vi "main.vi"() -> ()   [LabVIEW 2012]
uses:
  <userlib>/atmcd32d.llb/Error Code Enum typedef.ctl
  <userlib>/atmcd32d.llb/AcquisitionMode_mode typedef.ctl
  <userlib>/atmcd32d.llb/Spool_method typedef.ctl
  <vilib>/Analysis/NI_AALBase.lvlib
panel:
  in  "Analysis":bool
  in  "Scan":bool
  in  "MotorMgr":bool
  in  "sub_img_width":u16=9 min=5 max=511 step=2
  out "hist max":dbl
  out "hist min":dbl
  in  "hist_auto":bool=TRUE caption="auto"
  in  "hist_reset":bool
  in  "hist_set":cluster{u16, u16}(slide)={0, 502} scale=591.0..843.0
  out "histogram":T1(graph)
  out "sub_image":i32[][](graph)
  in  "reset ROI":bool
  in  "ROI":bool
  out "LastMousePos":cluster{"X":dbl, "Y":dbl}
  in  "disp_ye":u16=512 min=1 max=512 step=1
  in  "disp_xe":u16=512 min=1 max=512 step=1
  in  "disp_ys":u16=1 min=1 max=512 step=1
  in  "disp_xs":u16=1 min=1 max=512 step=1
  in  "Y_end":u16=512 min=1 max=512 step=1
  in  "X_end":u16=512 min=1 max=512 step=1
  in  "Y_start":u16=1 min=1 max=512 step=1
  in  "X_start":u16=1 min=1 max=512 step=1
  out "acq":bool
  out "video":bool
  out "error out":errorcluster
  in  "temp switch":bool
  out "temp status":T2
  out "temperature":i32
  out "kinetic":sgl format="%.2f"
  out "exposure":sgl format="%.2f"
  out "status":T2
  out "error out 2":errorcluster
  in  "close":bool
  out "sys on":bool
  out "frame":dbl
  in  "STOP":bool
  in  "A":bool
  in  "V":bool
  in  "Baseline Clamp":bool=TRUE
  in  "Path":path=path "e:/ipalm"
  in  "File Name":string="spool"
  in  "Kinetics Cycle Time":dbl
  in  "Frame Transfer":bool=TRUE
  in  "Aquisition Mode":u16(ring)=3 items=["Single"=1, "Kinetics"=3, "Fast Kinetics"=4]
  in  "Kinetics number":u32=1 min=1 step=1
  in  "Trigger Mode":u16(ring) items=["Internal"=0, "External"=1, "External Start"=6, "External Exposure"=7, "Software Trigger"=10]
  in  "温度":i32 min=-100 max=20 step=1
  in  "Exp Time":dbl(slide) min=0.0 scale=0.01..1.0
  in  "EM Gain":u16(slide)=1 min=1 max=300 step=1 scale=0.0..300.0
  out "强度图":i32[][](graph)
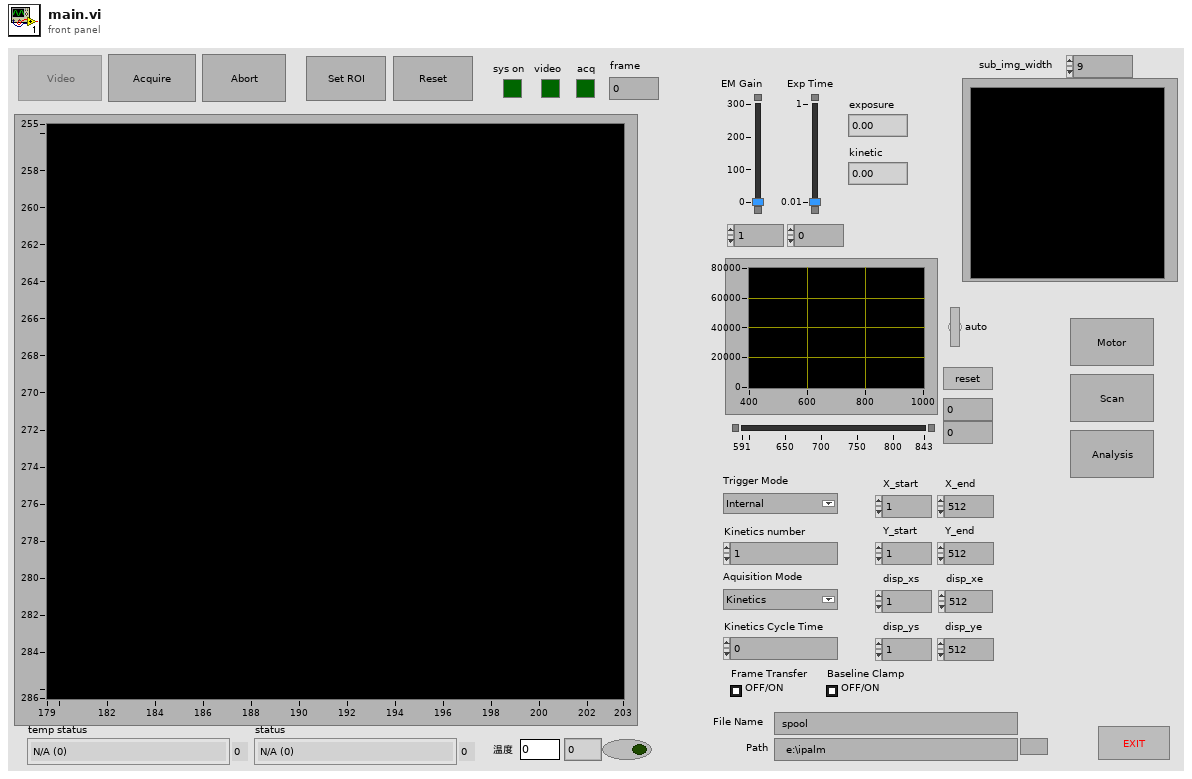
[diagram p1: front panel]
types:
  T1 = cluster{"X Values":dbl[], "Histogram: h(x)":i32[]}
  T2 = typedef "Error Code Enum typedef.ctl" = enum32{"N/A (0)", "DRV_ERROR_CODES", "DRV_SUCCESS", "DRV_VXDNOTINSTALLED", "DRV_ERROR_SCAN", "DRV_ERROR_CHECK_SUM", "DRV_ERROR_FILELOAD", "DRV_UNKNOWN_FUNC", "DRV_ERROR_VXD_INIT", "DRV_ERROR_ADDRESS", "DRV_ERROR_PAGELOCK", "DRV_ERROR_PAGEUNLOCK", "DRV_ERROR_BOARDTEST", "DRV_ERROR_ACK", "DRV_ERROR_UP_FIFO", "DRV_ERROR_PATTERN", "N/A (16)", "DRV_ACQUISITION_ERRORS", "DRV_ACQ_BUFFER", "DRV_ACQ_DOWNFIFO_FULL", "DRV_PROC_UNKONWN_INSTRUCTION", "DRV_ILLEGAL_OP_CODE", "DRV_KINETIC_TIME_NOT_MET", "DRV_ACCUM_TIME_NOT_MET", "DRV_NO_NEW_DATA", "N/A (25)", "DRV_SPOOLERROR", "N/A (27)", "N/A (28)", "N/A (29)", "N/A (30)", "N/A (31)", "N/A (32)", "DRV_TEMPERATURE_CODES", "DRV_TEMPERATURE_OFF", "DRV_TEMPERATURE_NOT_STABILIZED", "DRV_TEMPERATURE_STABILIZED", "DRV_TEMPERATURE_NOT_REACHED", "DRV_TEMPERATURE_OUT_RANGE", "DRV_TEMPERATURE_NOT_SUPPORTED", "DRV_TEMPERATURE_DRIFT", "N/A (41)", "N/A (42)", "N/A (43)", "N/A (44)", "N/A (45)", "N/A (46)", "N/A (47)", "N/A (48)", "DRV_GENERAL_ERRORS", "DRV_INVALID_AUX", "DRV_COF_NOTLOADED", "DRV_FPGAPROG", "DRV_FLEXERROR", "DRV_GPIBERROR", "N/A (55)", "N/A (56)", "N/A (57)", "N/A (58)", "N/A (59)", "N/A (60)", "N/A (61)", "N/A (62)", "N/A (63)", "DRV_DATATYPE", "DRV_DRIVER_ERRORS", "DRV_P1INVALID", "DRV_P2INVALID", "DRV_P3INVALID", "DRV_P4INVALID", "DRV_INIERROR", "DRV_COFERROR", "DRV_ACQUIRING", "DRV_IDLE", "DRV_TEMPCYCLE", "DRV_NOT_INITIALIZED", "DRV_P5INVALID", "DRV_P6INVALID", "DRV_INVALID_MODE", "DRV_INVALID_FILTER", "DRV_I2CERRORS", "DRV_I2CDEVNOTFOUND", "DRV_I2CTIMEOUT", "DRV_P7INVALID", "N/A (84)", "N/A (85)", "N/A (86)", "N/A (87)", "N/A (88)", "N/A (89)", "DRV_IOCERROR", "DRV_VRMVERSIONERROR"}
  T3 = cluster{"X_start":u16, "X_end":u16, "Y_start":u16, "Y_end":u16}
  T4 = cluster{"X_start":bool, "X_end":bool, "Y_start":bool, "Y_end":bool}
  T5 = cluster{"hist_set":cluster{u16, u16}, "hist_reset":bool, "hist_auto":bool, "Value":dbl, "Value":dbl}
  T6 = cluster{"hist_set":cluster{bool, bool}, "hist_reset":bool, "hist_auto":bool, "Value":bool, "Value":bool}
  T7 = cluster{"image":i16[][], "x_start":u32, "x_end":u32, "y_start":u32, "y_end":u32, "ImageCnt":u32, "subImage":u16[][]}
  T8 = typedef "AcquisitionMode_mode typedef.ctl" = enum16{"Reserved (0)", "Single Scan", "Accumulate", "Kinetics", "Fast Kinetics", "Run Till Abort", "Reserved (6)", "Reserved (7)", "Reserved (8)", "Time Delayed Integration"}
  T9 = typedef "Spool_method typedef.ctl" = enum16{"32-bit", "Depends", "16-bit", "Multiple Directory", "Spool to RAM disk", "16-bit FITS", "SIF", "16-buit TIFF", "Multiple Directory Compressed"}
  T10 = enum32{"Invalid", "Standard", "Closed", "Hidden", "Minimized", "Maximized"}
  T11 = typedef "LVPoint32TypeDef.ctl" = cluster{"Horizontal":i32, "Vertical":i32}
  T12 = cluster{"Position":cluster{"X":dbl, "Y":dbl}, "DoubleClick":bool}
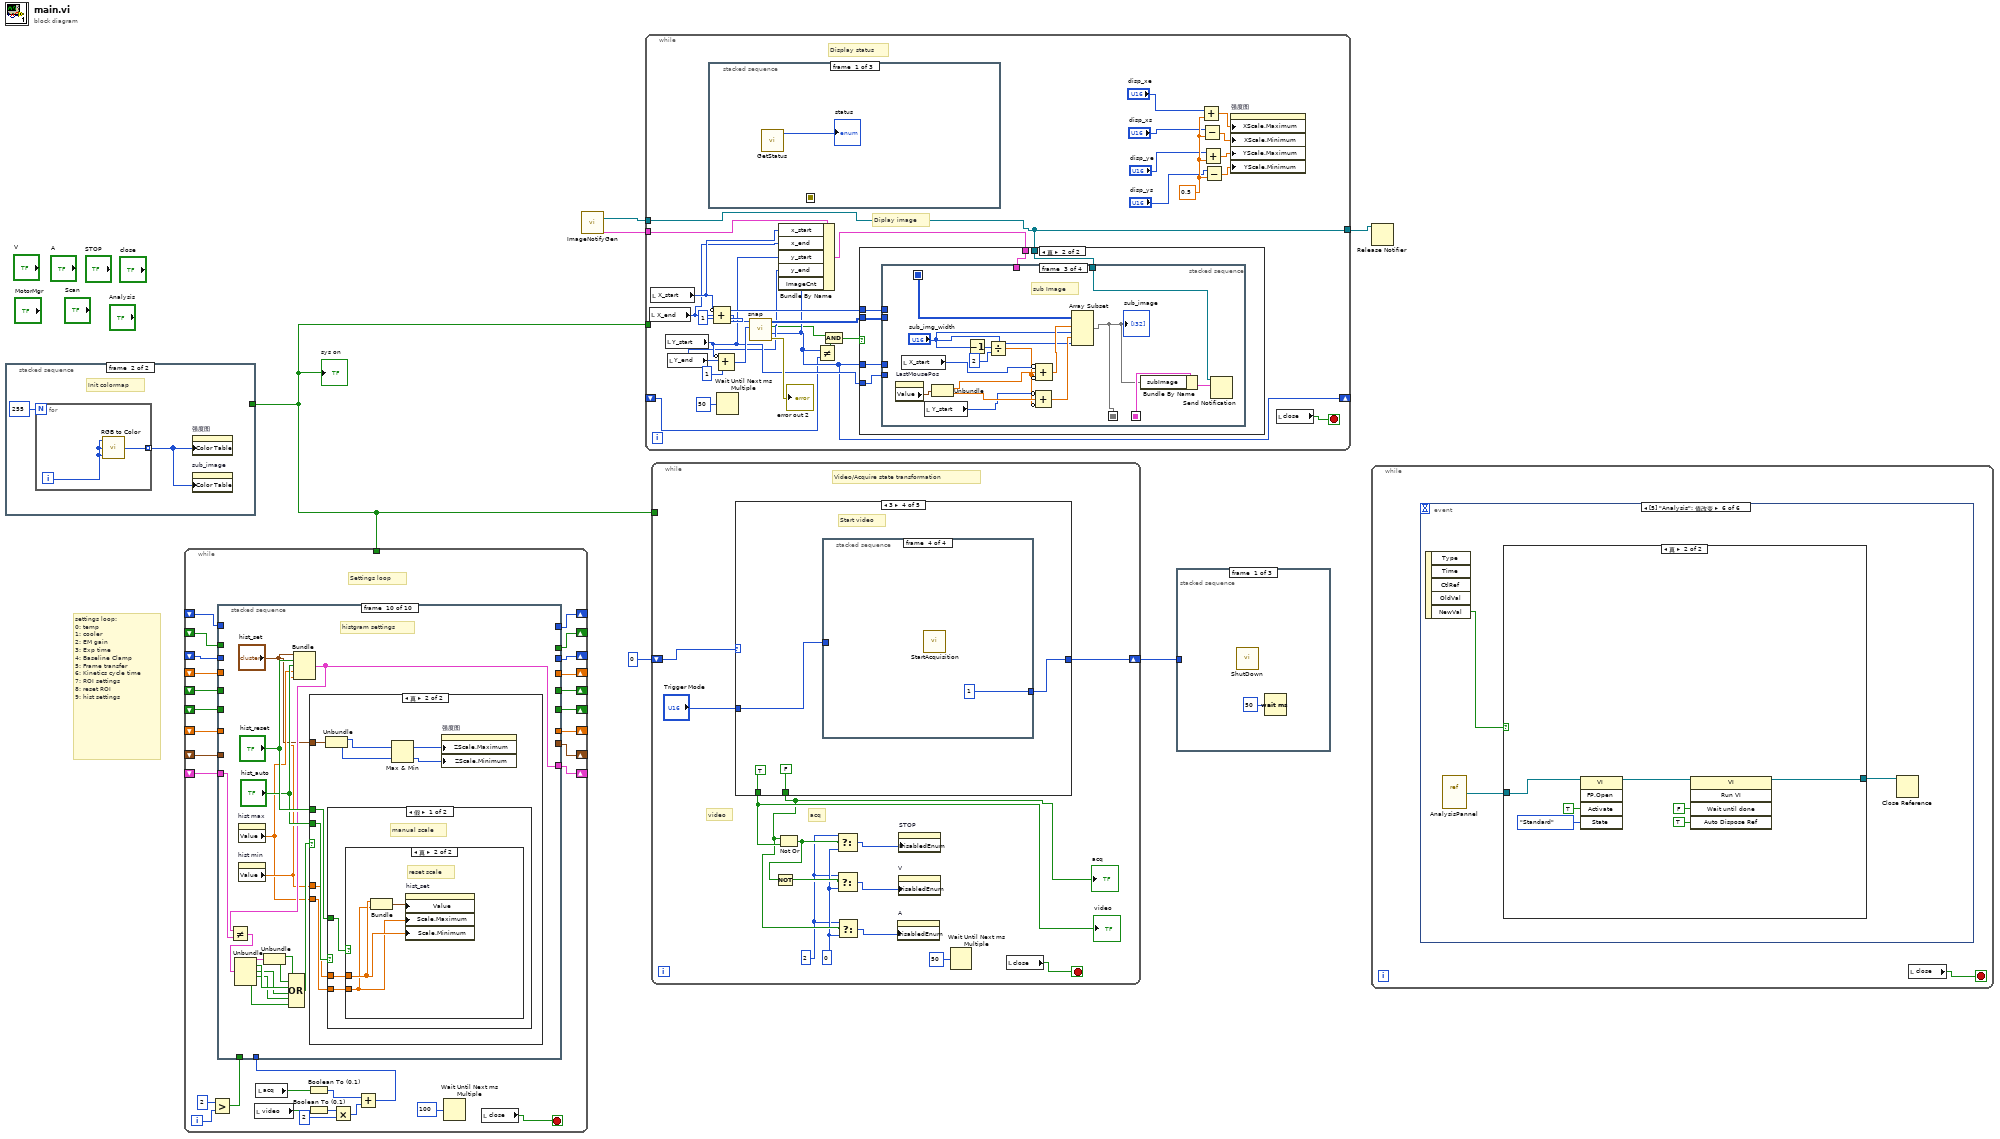
[diagram p0: block diagram]
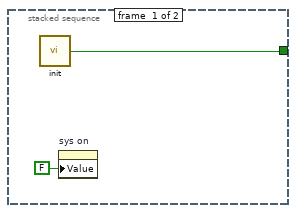
[diagram p2: hidden frame]
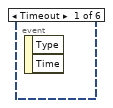
[diagram p3: hidden frame]
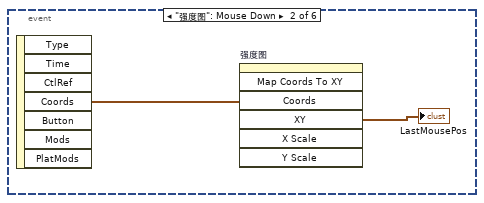
[diagram p4: hidden frame]
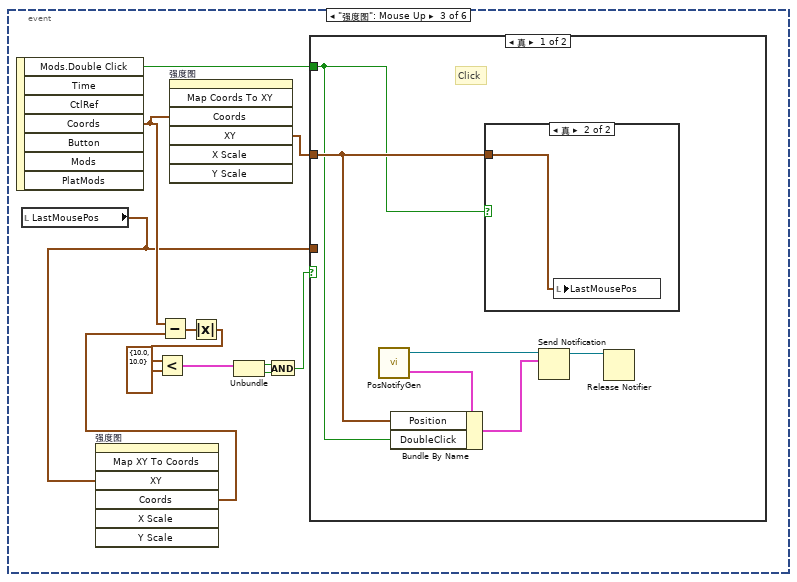
[diagram p5: hidden frame]
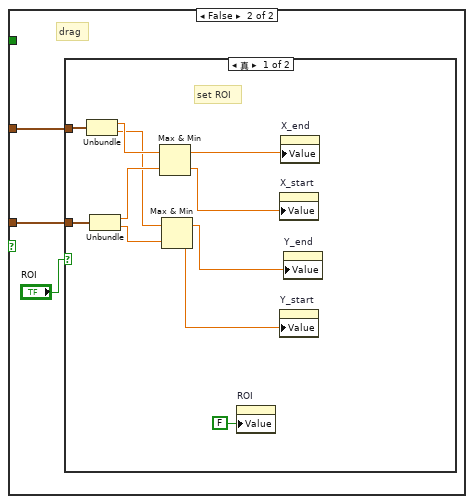
[diagram p7: hidden frame]
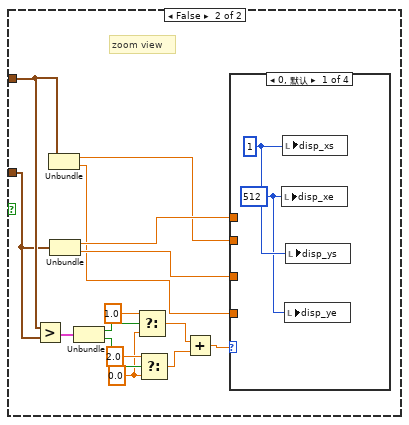
[diagram p8: hidden frame]
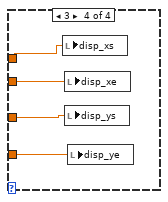
[diagram p11: hidden frame]
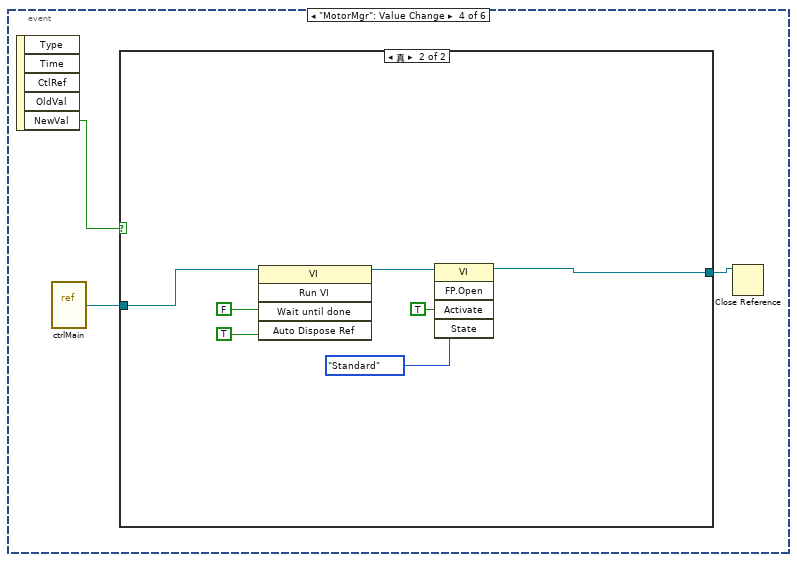
[diagram p12: hidden frame]
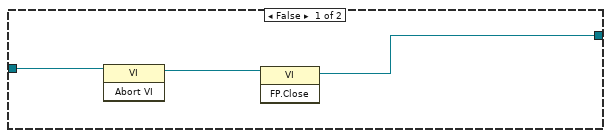
[diagram p13: hidden frame]
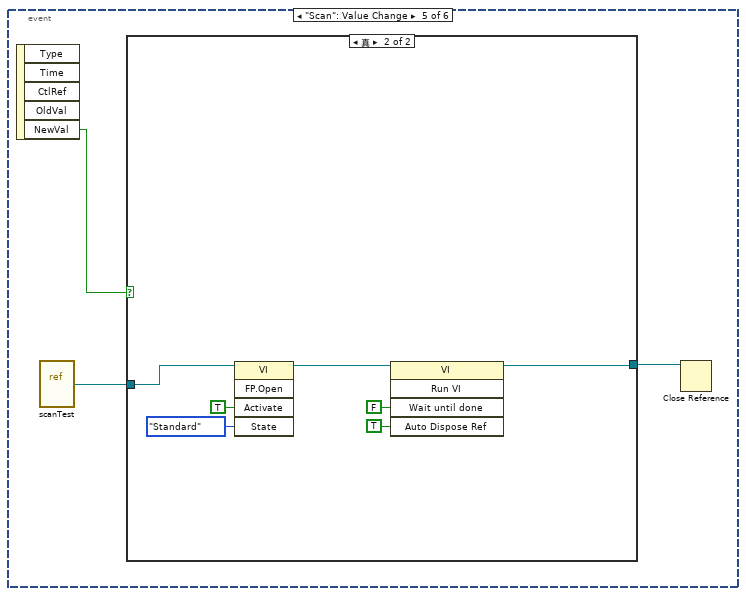
[diagram p14: hidden frame]
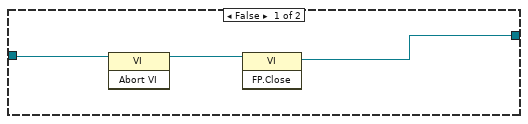
[diagram p15: hidden frame]
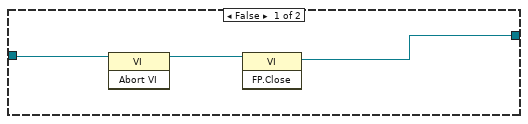
[diagram p16: hidden frame]
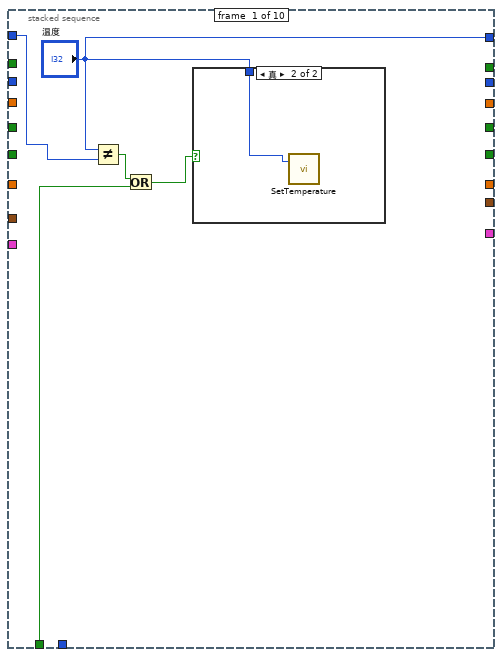
[diagram p17: hidden frame]
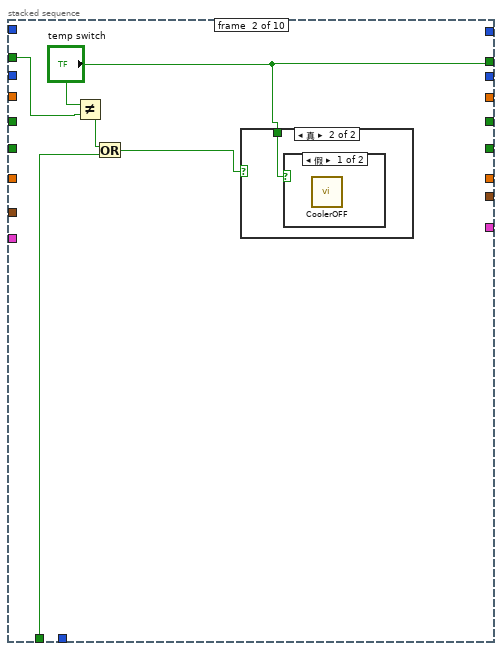
[diagram p19: hidden frame]
diagram:
  # "settings loop:\n0: temp\n1: cooler\n2: EM gain\n3: Exp time\n4: Baseline Clamp\n5: Frame transfer\n6: Kinetics cycle time\n7: ROI settings\n8: reset ROI\n9: hist settings"
  n1 = stacked-sequence {
    tunnel: [w8 _] -> w4
    frame #0 {
      n2 = call "init.vi"() -> ("success"=w8:bool)  [unwired: 1 in]
      n3 = property on="sys on" class="Bool (严格)"("Value"=FALSE ("system on")) -> ()  [unwired: 2 in, 2 out]
    }
    frame #1 {
      # "Init colormap"
      n4 = for {
        N: 255 -> [_]
        tunnel: [w12] -> w9 mode=indexing
        i -> [w11]
        n5 = call <vilib>:"RGB to Color.vi"("B"=w11, "G"=w11, "R"=w11) -> ("Color"=w12:u32)
      }
      n6 = property on="强度图" class="IntGraph (严格)"("Color Table"=w9) -> ()  [unwired: 2 in, 2 out]
      n7 = property on="sub_image" class="IntGraph (严格)"("Color Table"=w9) -> ()  [unwired: 2 in, 2 out]
    }
  }
  "sys on" <- w4
  n8 = while {
    shift-right: [w40] -> _
    shift-left: _ -> [w39]
    shift-right: [w38] -> _
    shift-left: _ -> [w37]
    shift-right: [w36] -> _
    shift-left: _ -> [w35]
    shift-right: [w34] -> _
    shift-left: _ -> [w33]
    shift-right: [w32] -> _
    shift-left: _ -> [w31]
    shift-right: [w30] -> _
    shift-left: _ -> [w29]
    shift-right: [w28] -> _
    shift-left: _ -> [w27]
    tunnel: w4 -> [_]
    shift-right: [w16] -> _
    shift-left: _ -> [w15]
    shift-right: [w14] -> _
    shift-left: _ -> [w13]
    i -> [w25]
    stop <- w42 stop-if-true
    # "Settings loop"
    n9 = Greater?(x=2, y=w25) -> (0:w24:bool)
    n10 = local read "video"() -> (w22:bool)
    n11 = local read "acq"() -> (w23:bool)
    n12 = Boolean To (0,1)(Boolean=w23) -> (0, 1=w18:i16)
    n13 = Boolean To (0,1)(Boolean=w22) -> (0, 1=w21:i16)
    n14 = Multiply(x=w21, y=i16 2) -> (x*y=w19:i16)
    n15 = Add(x=w18, y=w19) -> (x+y=w17:i16)
    n16 = stacked-sequence {
      tunnel: ["温度" _ _ _ _ _ _ _ _ _] -> w40
      tunnel: w39 -> [w47 _ _ _ _ _ _ _ _ _]
      tunnel: [_ "temp switch" _ _ _ _ _ _ _ _] -> w38
      tunnel: w37 -> [_ w53 _ _ _ _ _ _ _ _]
      tunnel: [_ _ "EM Gain" _ _ _ _ _ _ _] -> w36
      tunnel: w35 -> [_ _ w60 _ _ _ _ _ _ _]
      tunnel: [_ _ _ "Exp Time" _ _ _ _ _ _] -> w34
      tunnel: w33 -> [_ _ _ w71 _ _ _ _ _ _]
      tunnel: [_ _ _ _ "Baseline Clamp" _ _ _ _ _] -> w32
      tunnel: w31 -> [_ _ _ _ w82 _ _ _ _ _]
      tunnel: [_ _ _ _ _ "Frame Transfer" _ _ _ _] -> w30
      tunnel: w29 -> [_ _ _ _ _ w92 _ _ _ _]
      tunnel: [_ _ _ _ _ _ "Kinetics Cycle Time" _ _ _] -> w28
      tunnel: w27 -> [_ _ _ _ _ _ w104 _ _ _]
      tunnel: w24 -> [w44 w50 w57 w69 w79 w90 w102 _ _ _]
      tunnel: w17 -> [_ _ w55 w67 w77 w88 w100 w111 _ _]
      tunnel: [_ _ _ _ _ _ _ w112 _ _] -> w16
      tunnel: w15 -> [_ _ _ _ _ _ _ w119 _ _]
      tunnel: [_ _ _ _ _ _ _ _ _ w157] -> w14
      tunnel: w13 -> [_ _ _ _ _ _ _ _ _ w162]
      frame #0 {
        n17 = Not Equal?(x="温度", y=w47) -> (x != y?=w45:bool)
        n18 = Or(x=w45, y=w44) -> (x .or. y?=w43:bool)
        n19 = case shown="真" w43 {
          tunnel: "温度" -> [_ w48]
          frame False {
          }
          frame True {
            n20 = call <userlib>:"SetTemperature.vi"("temperature"=w48) -> ()  [unwired: 1 in, 2 out]
          }
        }
      }
      frame #1 {
        n21 = Not Equal?(x="temp switch", y=w53) -> (x != y?=w51:bool)
        n22 = Or(x=w51, y=w50) -> (x .or. y?=w49:bool)
        n23 = case shown="真" w49 {
          tunnel: "temp switch" -> [_ w54]
          frame False {
          }
          frame True {
            n24 = case shown="假" w54 {
              frame False {
                n25 = call <userlib>:"CoolerOFF.vi"() -> ()  [unwired: 2 in, 2 out]
              }
              frame True {
                n26 = call <userlib>:"CoolerON.vi"() -> ()  [unwired: 2 in, 2 out]
              }
            }
          }
        }
      }
      frame #2 {
        n27 = Not Equal?(x="EM Gain", y=w60) -> (x != y?=w58:bool)
        n28 = Or(x=w58, y=w57) -> (x .or. y?=w56:bool)
        n29 = case shown="真" w56 {
          tunnel: "EM Gain" -> [_ w62]
          tunnel: w55 -> [_ w61]
          frame False {
          }
          frame True {
            n30 = case shown="2" w61 {
              tunnel: w62 -> [w63 _ w64]
              frame 0, Default {
                # "IDLE"
                n31 = call <userlib>:"SetEMCCDGain.vi"("gain"=w63) -> ()  [unwired: 1 in, 2 out]
              }
              frame 1 {
                # "acquisition"
              }
              frame 2 {
                # "video"
                n32 = stacked-sequence {
                  tunnel: w64 -> [_ w65 _]
                  frame #0 {
                    n33 = call <userlib>:"AbortAcquisition.vi"() -> ()  [unwired: 2 in, 2 out]
                  }
                  frame #1 {
                    n34 = call <userlib>:"SetEMCCDGain.vi"("gain"=w65) -> ()  [unwired: 1 in, 2 out]
                  }
                  frame #2 {
                    n35 = call <userlib>:"StartAcquisition.vi"() -> ()  [unwired: 2 in, 2 out]
                  }
                }
              }
            }
          }
        }
      }
      frame #3 {
        n36 = Not Equal?(x="Exp Time", y=w71) -> (x != y?=w68:bool)
        n37 = Or(x=w68, y=w69) -> (x .or. y?=w66:bool)
        n38 = case shown="真" w66 {
          tunnel: "Exp Time" -> [_ w73]
          tunnel: w67 -> [_ w72]
          frame False {
          }
          frame True {
            n39 = case shown="0, 默认" w72 {
              tunnel: w73 -> [w74 _ w75]
              frame 0, Default {
                # "IDLE"
                n40 = call <userlib>:"SetExposureTime.vi"("time"=w74) -> ()  [unwired: 1 in, 2 out]
              }
              frame 1 {
                # "acq"
              }
              frame 2 {
                # "video"
                n41 = stacked-sequence {
                  tunnel: w75 -> [_ w76 _]
                  frame #0 {
                    n42 = call <userlib>:"AbortAcquisition.vi"() -> ()  [unwired: 2 in, 2 out]
                  }
                  frame #1 {
                    n43 = call <userlib>:"SetExposureTime.vi"("time"=w76) -> ()  [unwired: 1 in, 2 out]
                  }
                  frame #2 {
                    n44 = call <userlib>:"StartAcquisition.vi"() -> ()  [unwired: 2 in, 2 out]
                  }
                }
              }
            }
          }
        }
      }
      frame #4 {
        n45 = Not Equal?(x="Baseline Clamp", y=w82) -> (x != y?=w80:bool)
        n46 = Or(x=w80, y=w79) -> (x .or. y?=w78:bool)
        n47 = case shown="真" w78 {
          tunnel: "Baseline Clamp" -> [_ w84]
          tunnel: w77 -> [_ w83]
          frame False {
          }
          frame True {
            n48 = case shown="0, 默认" w83 {
              tunnel: w84 -> [w85 _ w86]
              frame 0, Default {
                n49 = call <userlib>:"SetBaselineClamp.vi"("state"=w85) -> ()  [unwired: 1 in, 2 out]
              }
              frame 1 {
              }
              frame 2 {
                n50 = stacked-sequence {
                  tunnel: w86 -> [_ w87 _]
                  frame #0 {
                    n51 = call <userlib>:"AbortAcquisition.vi"() -> ()  [unwired: 2 in, 2 out]
                  }
                  frame #1 {
                    n52 = call <userlib>:"SetBaselineClamp.vi"("state"=w87) -> ()  [unwired: 1 in, 2 out]
                  }
                  frame #2 {
                    n53 = call <userlib>:"StartAcquisition.vi"() -> ()  [unwired: 2 in, 2 out]
                  }
                }
              }
            }
          }
        }
      }
      frame #5 {
        n54 = Not Equal?(x="Frame Transfer", y=w92) -> (x != y?=w91:bool)
        n55 = Or(x=w91, y=w90) -> (x .or. y?=w89:bool)
        n56 = case shown="真" w89 {
          tunnel: "Frame Transfer" -> [_ w95]
          tunnel: w88 -> [_ w94]
          frame False {
          }
          frame True {
            n57 = Boolean To (0,1)(Boolean=w95) -> (0, 1=w96:i16)
            n58 = case shown="0, 默认" w94 {
              tunnel: w96 -> [w97 _ w98]
              frame 0, Default {
                n59 = call <userlib>:"SetFrameTransferMode.vi"("mode"=w97) -> ()  [unwired: 1 in, 2 out]
              }
              frame 1 {
              }
              frame 2 {
                n60 = stacked-sequence {
                  tunnel: w98 -> [_ w99 _]
                  frame #0 {
                    n61 = call <userlib>:"AbortAcquisition.vi"() -> ()  [unwired: 2 in, 2 out]
                  }
                  frame #1 {
                    n62 = call <userlib>:"SetFrameTransferMode.vi"("mode"=w99) -> ()  [unwired: 1 in, 2 out]
                  }
                  frame #2 {
                    n63 = call <userlib>:"StartAcquisition.vi"() -> ()  [unwired: 2 in, 2 out]
                  }
                }
              }
            }
          }
        }
      }
      frame #6 {
        n64 = Not Equal?(x="Kinetics Cycle Time", y=w104) -> (x != y?=w103:bool)
        n65 = Or(x=w103, y=w102) -> (x .or. y?=w101:bool)
        n66 = case shown="真" w101 {
          tunnel: "Kinetics Cycle Time" -> [_ w107]
          tunnel: w100 -> [_ w106]
          frame False {
          }
          frame True {
            n67 = case shown="0, 默认" w106 {
              tunnel: w107 -> [w108 _ w109]
              frame 0, Default {
                n68 = call <userlib>:"SetKineticCycleTime.vi"("time"=w108) -> ()  [unwired: 1 in, 2 out]
              }
              frame 1 {
              }
              frame 2 {
                n69 = stacked-sequence {
                  tunnel: w109 -> [_ w110 _]
                  frame #0 {
                    n70 = call <userlib>:"AbortAcquisition.vi"() -> ()  [unwired: 2 in, 2 out]
                  }
                  frame #1 {
                    n71 = call <userlib>:"SetKineticCycleTime.vi"("time"=w110) -> ()  [unwired: 1 in, 2 out]
                  }
                  frame #2 {
                    n72 = call <userlib>:"StartAcquisition.vi"() -> ()  [unwired: 2 in, 2 out]
                  }
                }
              }
            }
          }
        }
      }
      frame #7 {
        # "ROI settings"
        n73 = Bundle("X_start"="X_start", "X_end"="X_end", "Y_start"="Y_start", "Y_end"="Y_end") -> (w112:T3)  [unwired: 1 in]
        n74 = Not Equal?(x=w112, y=w119) -> (x != y?=w118:T4)
        n75 = Unbundle(w118) -> ("X_start"=w117:bool, "X_end"=w115:bool, "Y_start"=w116:bool, "Y_end"=w114:bool)
        n76 = Compound Arithmetic op=OR(w117, w115, w116, w114) -> (w113:bool)
        n77 = case shown="真" w113 {
          tunnel: w112 -> [_ w129]
          tunnel: w111 -> [_ w128]
          frame False {
          }
          frame True {
            n78 = Unbundle(w129) -> ("X_start"=w127:u16, "X_end"=w126:u16, "Y_start"=w125:u16, "Y_end"=w124:u16)
            n79 = case shown="0, 默认" w128 {
              tunnel: w125 -> [w133 _ w138]
              tunnel: w124 -> [w132 _ w137]
              tunnel: w127 -> [w131 _ w136]
              tunnel: w126 -> [w130 _ w135]
              frame 0, Default {
                w134 = 1 ("hbin")
                n80 = call <userlib>:"SetImage.vi"("hbin"=w134, "vbin"=w134, "hstart"=w133, "hend"=w132, "vstart"=w131, "vend"=w130) -> ()  [unwired: 20 in, 2 out]
              }
              frame 1 {
              }
              frame 2 {
                n81 = stacked-sequence {
                  tunnel: w138 -> [_ w142 _]
                  tunnel: w137 -> [_ w141 _]
                  tunnel: w136 -> [_ w140 _]
                  tunnel: w135 -> [_ w139 _]
                  frame #0 {
                    n82 = call <userlib>:"AbortAcquisition.vi"() -> ()  [unwired: 2 in, 2 out]
                  }
                  frame #1 {
                    w143 = 1 ("hbin")
                    n83 = call <userlib>:"SetImage.vi"("hbin"=w143, "vbin"=w143, "hstart"=w142, "hend"=w141, "vstart"=w140, "vend"=w139) -> ()  [unwired: 20 in, 2 out]
                  }
                  frame #2 {
                    n84 = call <userlib>:"StartAcquisition.vi"() -> ()  [unwired: 2 in, 2 out]
                  }
                }
              }
            }
          }
        }
      }
      frame #8 {
        # "reset ROI"
        n85 = case shown="真" "reset ROI" {
          frame False {
          }
          frame True {
            w145 = u16 512 ("X_end")
            w146 = u16 1 ("X_start")
            n86 = property on="X_start" class="DigNum (严格)"("Value"=w146) -> ()  [unwired: 2 in, 2 out]
            n87 = property on="Y_start" class="DigNum (严格)"("Value"=w146) -> ()  [unwired: 2 in, 2 out]
            n88 = property on="X_end" class="DigNum (严格)"("Value"=w145) -> ()  [unwired: 2 in, 2 out]
            n89 = property on="Y_end" class="DigNum (严格)"("Value"=w145) -> ()  [unwired: 2 in, 2 out]
          }
        }
      }
      frame #9 {
        # "histgram settings"
        n90 = property on="hist max" class="DigNum (严格)"() -> ("Value"=w155:dbl)  [unwired: 2 in, 2 out]
        n91 = property on="hist min" class="DigNum (严格)"() -> ("Value"=w156:dbl)  [unwired: 2 in, 2 out]
        n92 = Bundle("hist_set"="hist_set", "hist_reset"="hist_reset", "hist_auto"="hist_auto", "Value"=w155, "Value"=w156) -> (w157:T5)  [unwired: 1 in]
        n93 = Not Equal?(x=w157, y=w162) -> (x != y?=w161:T6)
        n94 = Unbundle(w161) -> ("hist_set"=w153:cluster{bool, bool}, "hist_reset"=w150:bool, "hist_auto"=w149:bool, "Value"=w148:bool, "Value"=w147:bool)
        n95 = Unbundle(w153) -> (w152:bool, w151:bool)
        n96 = Compound Arithmetic op=OR(w152, w151, w150, w149, w148, w147) -> (w160:bool)
        n97 = case shown="真" w160 {
          tunnel: "hist_set" -> [_ w165]
          tunnel: "hist_reset" -> [_ w170]
          tunnel: "hist_auto" -> [_ w171]
          tunnel: w156 -> [_ w169]
          tunnel: w155 -> [_ w168]
          frame False {
          }
          frame True {
            n98 = Unbundle(w165) -> (w164:u16, w163:u16)
            n99 = case shown="假" w171 {
              tunnel: w170 -> [w174 _]
              tunnel: w169 -> [w173 w179]
              tunnel: w168 -> [w172 w178]
              frame False {
                # "manual scale"
                n100 = case shown="真" w174 {
                  tunnel: w173 -> [_ w176]
                  tunnel: w172 -> [_ w175]
                  frame False {
                    # "set scale"
                  }
                  frame True {
                    # "reset scale"
                    n101 = Bundle("Value"=w176, "Value"=w175) -> (w177:cluster{"Value":dbl, "Value":dbl})  [unwired: 1 in]
                    n102 = property on="hist_set" class="Slide (严格)"("Value"=w177, "Scale.Maximum"=w175, "Scale.Minimum"=w176) -> ()  [unwired: 2 in, 2 out]
                  }
                }
              }
              frame True {
                # "Auto scale"
                n103 = Bundle("Value"=w179, "Value"=w178) -> (w180:cluster{"Value":dbl, "Value":dbl})  [unwired: 1 in]
                n104 = property on="hist_set" class="Slide (严格)"("Scale.Maximum"=w178, "Scale.Minimum"=w179, "Value"=w180) -> ()  [unwired: 2 in, 2 out]
              }
            }
            n105 = Max & Min(x=w164, y=w163) -> (max(x,y)=w167:u16, min(x,y)=w166:u16)
            n106 = property on="强度图" class="IntGraph (严格)"("ZScale.Maximum"=w167, "ZScale.Minimum"=w166) -> ()  [unwired: 2 in, 2 out]
          }
        }
      }
    }
    n107 = Wait Until Next ms Multiple(millisecond multiple=u32 100 ("毫秒倍数")) -> ()  [unwired: 1 out]
    n108 = local read "close"() -> (w42:bool)
  }
  n109 = call "ImageNotifyGen.vi"() -> ("ImageClusterRef"=w2:T7, "ImageNotifyRef"=w3:refnum<notifier>)  [unwired: 2 in]
  n110 = while {
    tunnel: w4 -> [_]
    tunnel: w3 -> [w186]
    tunnel: w2 -> [w187]
    tunnel: [w186] -> w1
    shift-right: [w185] -> _
    shift-left: _ -> [w184]
    stop <- w208 stop-if-true
    w201 = 0.5 ("y")
    # "Diplay image"
    # "Display status"
    n111 = local read "X_end"() -> (w191:u16)
    n112 = local read "X_start"() -> (w192:u16)
    n113 = local read "Y_start"() -> (w190:u16)
    n114 = local read "Y_end"() -> (w189:u16)
    n115 = stacked-sequence {
      seq-local: [_ w211 _] -> [_ _ w215]
      frame #0 {
        n116 = call <userlib>:"GetStatus.vi"() -> ("status"=→"status":T2)  [unwired: 3 in, 2 out]
      }
      frame #1 {
        n117 = call <userlib>:"GetAcquisitionTimings.vi"() -> ("exposure"=→"exposure":sgl, "kinetic"=→"kinetic":sgl, "error out"=w211:errorcluster)  [unwired: 11 in, 2 out]
      }
      frame #2 {
        n118 = call <userlib>:"GetTemperature.vi"("error in (no error)"=w215) -> ("error out"=→"error out":errorcluster, "status"=→"temp status":T2, "temperature"=→"temperature":i32)  [unwired: 3 in, 1 out]
      }
    }
    n119 = Compound Arithmetic op=ADD(invert w192, w191, u16 1 ("值")) -> (w204:u16)
    n120 = Wait Until Next ms Multiple(millisecond multiple=u32 50 ("毫秒倍数")) -> ()  [unwired: 1 out]
    n121 = Compound Arithmetic op=ADD(invert w190, w189, u16 1 ("值")) -> (w203:u16)
    n122 = call "snap.vi"("y"=w203, "x"=w204) -> ("error out 2"=→"error out 2":errorcluster, "ImgCnt"=w185:i32, "Valid"=w182:bool, "Image"=w202:i32[][])  [unwired: 2 in]
    n123 = Bundle By Name(cluster=w187, "x_start"=w192, "x_end"=w191, "y_start"=w190, "y_end"=w189, "ImageCnt"=w185) -> (w188:T7)
    n124 = Not Equal?(x=w185, y=w184) -> (x != y?=w183:bool)
    n125 = And(x=w182, y=w183) -> (x .and. y?=w181:bool)
    n126 = case shown="真" w181 {
      tunnel: w202 -> [_ w223]
      tunnel: w185 -> [_ w222]
      tunnel: w190 -> [_ w220]
      tunnel: w192 -> [_ w221]
      tunnel: w188 -> [_ w219]
      tunnel: w186 -> [_ w218]
      frame False {
      }
      frame True {
        n127 = stacked-sequence {
          seq-local: [w225 _ _ _] -> [_ _ w247 w259]
          seq-local: [_ _ w239 _] -> [_ _ _ _]
          seq-local: [w224 _ _ _] -> [_ _ w240 _]
          tunnel: w223 -> [w225 _ _ _]
          tunnel: w222 -> [w227 _ _ _]
          tunnel: w221 -> [_ w229 _ _]
          tunnel: w220 -> [_ w230 _ _]
          tunnel: w219 -> [w226 _ _ _]
          tunnel: w218 -> [_ _ w238 _]
          frame #0 {
            n128 = Bundle By Name(cluster=w226, "image"=w225) -> (w224:T7)
            "强度图" <- w225
            "frame" <- w227
          }
          frame #1 {
            w228 = 0.5 ("y")
            n129 = Subtract(x=w230, y=w228) -> (x-y=w231:dbl)
            n130 = Subtract(x=w229, y=w228) -> (x-y=w232:dbl)
            n131 = property on="强度图" class="IntGraph (严格)"("XScale.Offset"=w232) -> ()  [unwired: 2 in, 2 out]
            n132 = property on="强度图" class="IntGraph (严格)"("YScale.Offset"=w231) -> ()  [unwired: 2 in, 2 out]
          }
          frame #2 {
            # "sub Image"
            n133 = property on="LastMousePos" class="Clust (严格)"() -> ("Value"=w248:cluster{"X":dbl, "Y":dbl})  [unwired: 2 in, 2 out]
            n134 = local read "X_start"() -> (w242:u16)
            n135 = local read "Y_start"() -> (w241:u16)
            n136 = Unbundle(w248) -> ("X"=w246:dbl, "Y"=w245:dbl)
            n137 = Decrement(x="sub_img_width") -> (x-1=w235:u16)
            n138 = Divide(x=w235, y=u16 2) -> (x/y=w233:dbl)
            n139 = Compound Arithmetic op=ADD(invert w241, w245, invert w233) -> (w243:dbl)
            n140 = Compound Arithmetic op=ADD(invert w242, w246, invert w233) -> (w244:dbl)
            n141 = Array Subset(array=w247, index (row)=w244, length (row)="sub_img_width", index (col)=w243, length (col)="sub_img_width") -> (w239:i32[][])
            "sub_image" <- w239
            n142 = Bundle By Name(cluster=w240, "subImage"=w239) -> (w237:T7)
            n143 = Send Notification(notification=w237, notifier=w238) -> ()  [unwired: 1 in, 2 out]
          }
          frame #3 {
            n144 = Array Size(array=w259) -> (size(s)=w257:i32[])
            n145 = Index Array(array=w257, index=0 ("索引")) -> (element=w255:i32)
            n146 = Index Array(array=w257, index=1 ("索引")) -> (element=w254:i32)
            n147 = Multiply(x=w255, y=w254) -> (x*y=w253:i32)
            n148 = Reshape Array(w259, w253) -> (w251:i32[])
            n149 = call <vilib>:"Histogram.vi"("intervals"=20, "X"=w251) -> ("Histogram Graph"=→"histogram":T1)  [unwired: 6 in, 3 out]
            n150 = Array Max & Min(array=w251) -> (max value=→"hist max":i32, min value=→"hist min":i32)  [unwired: 2 out]
          }
        }
      }
    }
    n151 = Add(x="disp_xe", y=w201) -> (x+y=w193:dbl)
    n152 = Subtract(x="disp_xs", y=w201) -> (x-y=w194:dbl)
    n153 = Add(x="disp_ye", y=w201) -> (x+y=w195:dbl)
    n154 = Subtract(x="disp_ys", y=w201) -> (x-y=w196:dbl)
    n155 = property on="强度图" class="IntGraph (严格)"("XScale.Maximum"=w193, "XScale.Minimum"=w194, "YScale.Maximum"=w195, "YScale.Minimum"=w196) -> ()  [unwired: 2 in, 2 out]
    n156 = local read "close"() -> (w208:bool)
  }
  n157 = while {
    tunnel: w4 -> [_]
    shift-right: [w270] -> w5
    shift-left: 0 -> [w274]
    stop <- w271 stop-if-true
    w262 = i16 0 ("f")
    w261 = i16 2 ("t")
    # "acq"
    # "video"
    # "Video/Acquire state transformation"
    n158 = case shown="3" w274 {
      tunnel: [w276 w293 w299 w308 w319] -> w270
      tunnel: "Trigger Mode" -> [_ _ _ w309 w320]
      tunnel: [w275 FALSE TRUE FALSE TRUE] -> w266
      tunnel: [w275 TRUE FALSE TRUE FALSE] -> w269
      frame 0, Default {
        w275 = FALSE
        # "IDLE wait for video or acquisition"
        n159 = local read "A"() -> (w281:bool)
        n160 = local read "V"() -> (w283:bool)
        n161 = Or(x=w281, y=w283) -> (x .or. y?=w282:bool)
        n162 = Select(t=i8 4 ("f"), s=w281, f=i8 3) -> (s? t:f=w277:i8)
        n163 = Select(t=w277, s=w282, f=i8 0) -> (s? t:f=w276:i8)
      }
      frame 1 {
        # "Video mode"
        n164 = local read "A"() -> (w285:bool)
        n165 = local read "STOP"() -> (w284:bool)
        n166 = Or(x=w285, y=w284) -> (x .or. y?=w286:bool)
        n167 = case shown="真" w286 {
          frame False {
          }
          frame True {
            n168 = stacked-sequence {
              frame #0 {
                n169 = call <userlib>:"AbortAcquisition.vi"() -> ()  [unwired: 2 in, 2 out]
              }
              frame #1 {
                w294 = FALSE ("STOP")
                n170 = local write "STOP"(w294) -> ()
                n171 = local write "A"(w294) -> ()
              }
            }
          }
        }
        n172 = Select(t=i8 4, s=w285, f=i8 1 ("t")) -> (s? t:f=w287:i8)
        n173 = Select(t=i8 0, s=w284, f=w287) -> (s? t:f=w293:i8)
      }
      frame 2 {
        # "Acquisition mode"
        n174 = call <userlib>:"GetStatus.vi"() -> ("status"=w304:T2)  [unwired: 3 in, 2 out]
        n175 = local read "STOP"() -> (w298:bool)
        n176 = Not Equal?(x=Error_Code_Enum_typedef."DRV_ACQUIRING", y=w304) -> (x != y?=w302:bool)
        n177 = case shown="真" w298 {
          frame False {
          }
          frame True {
            n178 = stacked-sequence {
              frame #0 {
                n179 = call <userlib>:"AbortAcquisition.vi"() -> ()  [unwired: 2 in, 2 out]
              }
              frame #1 {
                n180 = local write "STOP"(FALSE ("STOP")) -> ()
              }
            }
          }
        }
        n181 = Or(x=w302, y=w298) -> (x .or. y?=w301:bool)
        n182 = Select(t=i8 0, s=w301, f=i8 2) -> (s? t:f=w299:i8)
      }
      frame 3 {
        # "Start video"
        n183 = stacked-sequence {
          tunnel: w309 -> [_ w312 _ _]
          tunnel: [_ _ _ i8 1 ("f")] -> w308
          frame #0 {
            n184 = local write "V"(FALSE ("V")) -> ()
            n185 = call <userlib>:"SetAcquisitionMode.vi"("mode"=AcquisitionMode_mode_typedef."Run Till Abort") -> ()  [unwired: 1 in, 2 out]
          }
          frame #1 {
            n186 = call <userlib>:"SetTriggerMode.vi"("mode"=w312) -> ()  [unwired: 1 in, 2 out]
          }
          frame #2 {
            n187 = call <userlib>:"SetSpool.vi"("active"=FALSE, "method"=Spool_method_typedef."16-buit TIFF", "name"="") -> ()  [unwired: 11 in, 2 out]
          }
          frame #3 {
            n188 = call <userlib>:"StartAcquisition.vi"() -> ()  [unwired: 2 in, 2 out]
          }
        }
      }
      frame 4 {
        # "Start acquisition"
        n189 = stacked-sequence {
          tunnel: w320 -> [_ w322 _ _ _]
          tunnel: [_ _ _ _ i8 2 ("f")] -> w319
          frame #0 {
            n190 = call <userlib>:"SetAcquisitionMode.vi"("mode"="Aquisition Mode") -> ()  [unwired: 1 in, 2 out]
          }
          frame #1 {
            n191 = call <userlib>:"SetTriggerMode.vi"("mode"=w322) -> ()  [unwired: 1 in, 2 out]
          }
          frame #2 {
            n192 = call "path.vi"("file"="File Name", "path_in"="Path") -> ("path_out"=w323:string)
            n193 = call <userlib>:"SetSpool.vi"("active"=TRUE, "method"=Spool_method_typedef."16-buit TIFF", "name"=w323) -> ()  [unwired: 11 in, 2 out]
          }
          frame #3 {
            n194 = call <userlib>:"SetNumberKinetics.vi"("number"="Kinetics number") -> ()  [unwired: 1 in, 2 out]
          }
          frame #4 {
            n195 = local write "A"(FALSE ("A")) -> ()
            n196 = call <userlib>:"StartAcquisition.vi"() -> ()  [unwired: 2 in, 2 out]
          }
        }
      }
    }
    "video" <- w269
    "acq" <- w266
    n197 = Not Or(1:w269, 2:w266) -> (0:w268:bool)
    n198 = Not(x=w268) -> (.not. x?=w267:bool)
    n199 = Select(t=w261, s=w268, f=w262) -> (s? t:f=w265:i16)
    n200 = Select(t=w261, s=w267, f=w262) -> (s? t:f=w264:i16)
    n201 = Select(t=w261, s=w266, f=w262) -> (s? t:f=w263:i16)
    n202 = property on="A" class="Bool (严格)"("DisabledEnum"=w263) -> ()  [unwired: 2 in, 2 out]
    n203 = property on="V" class="Bool (严格)"("DisabledEnum"=w264) -> ()  [unwired: 2 in, 2 out]
    n204 = property on="STOP" class="Bool (严格)"("DisabledEnum"=w265) -> ()  [unwired: 2 in, 2 out]
    n205 = Wait Until Next ms Multiple(millisecond multiple=u32 50 ("毫秒倍数")) -> ()  [unwired: 1 out]
    n206 = local read "close"() -> (w271:bool)
  }
  n207 = stacked-sequence {
    tunnel: w5 -> [_ _ _]
    frame #0 {
      n208 = call <userlib>:"ShutDown.vi"() -> ()  [unwired: 2 in, 2 out]
      n209 = Wait (ms)(milliseconds to wait=u32 50 ("等待时间（毫秒）")) -> ()  [unwired: 1 out]
    }
    frame #1 {
      w332 = FALSE ("close")
      n210 = property on="sys on" class="Bool (严格)"("Value"=w332) -> ()  [unwired: 2 in, 2 out]
      n211 = local write "close"(w332) -> ()
    }
    frame #2 {
      n212 = Stop(stop? (T)=TRUE ("停止？(T)")) -> ()
    }
  }
  n213 = Release Notifier(notifier=w1) -> ()  [unwired: 2 in, 3 out]
  n214 = while {
    stop <- w334 stop-if-true
    n215 = event shown="[5] \"Analysis\": 值改变" {
      selector: _ -> [_ _ _ _ _ _]
      dyn-events: _ -> [_ _ _ _ _ _]
      timeout: _ -> [_ _ _ _ _ _]
      event Timeout {
        n216 = event-data() -> ()  [unwired: 1 in, 2 out]
      }
      event "强度图": Mouse Down {
        n217 = event-data() -> ("Coords"=w336:T11)  [unwired: 1 in, 6 out]
        n218 = invoke on="强度图" class="IntGraph (严格)" method="Map Coords To XY"("Coords"=w336) -> ("XY"=→"LastMousePos":cluster{"X":dbl, "Y":dbl})  [unwired: 6 in, 6 out]
      }
      event "强度图": Mouse Up {
        n219 = event-data() -> ("Mods.Double Click"=w337:bool, "Coords"=w340:T11)  [unwired: 1 in, 5 out]
        n220 = local read "LastMousePos"() -> (w339:cluster{"X":dbl, "Y":dbl})
        n221 = invoke on="强度图" class="IntGraph (严格)" method="Map XY To Coords"("XY"=w339) -> ("Coords"=w338:T11)  [unwired: 6 in, 6 out]
        n222 = Subtract(x=w340, y=w338) -> (x-y=w344:T11)
        n223 = invoke on="强度图" class="IntGraph (严格)" method="Map Coords To XY"("Coords"=w340) -> ("XY"=w348:cluster{"X":dbl, "Y":dbl})  [unwired: 6 in, 6 out]
        n224 = Absolute Value(x=w344) -> (abs(x)=w343:T11)
        n225 = Less?(x=w343, y=cluster{"X":dbl, "Y":dbl} {"X"=10.0, "Y"=10.0}) -> (x < y?=w341:cluster{bool, bool})
        n226 = Unbundle(w341) -> (w347:bool, w346:bool)
        n227 = And(x=w347, y=w346) -> (x .and. y?=w345:bool)
        n228 = case shown="真" w345 {
          tunnel: w348 -> [w351 w358]
          tunnel: w339 -> [_ w357]
          tunnel: w337 -> [w349 _]
          frame True {
            # "Click"
            n229 = call "PosNotifyGen.vi"() -> ("ClusterRef"=w352:T12, "NotifyRef"=w354:refnum<notifier>)  [unwired: 2 in]
            n230 = Bundle By Name(cluster=w352, "Position"=w351, "DoubleClick"=w349) -> (w350:T12)
            n231 = case shown="真" w349 {
              tunnel: w351 -> [_ w355]
              frame False {
              }
              frame True {
                n232 = local write "LastMousePos"(w355) -> ()
              }
            }
            n233 = Send Notification(notification=w350, notifier=w354) -> (notifier out=w353:refnum<notifier>)  [unwired: 1 in, 1 out]
            n234 = Release Notifier(notifier=w353) -> ()  [unwired: 2 in, 3 out]
          }
          frame False {
            # "drag"
            n235 = case shown="真" "ROI" {
              tunnel: w358 -> [w369 w371]
              tunnel: w357 -> [w368 w370]
              frame True {
                # "set ROI"
                n236 = Unbundle(w369) -> ("X"=w367:dbl, "Y"=w365:dbl)
                n237 = Unbundle(w368) -> ("X"=w366:dbl, "Y"=w364:dbl)
                n238 = Max & Min(x=w367, y=w366) -> (max(x,y)=w362:dbl, min(x,y)=w363:dbl)
                n239 = Max & Min(x=w365, y=w364) -> (max(x,y)=w361:dbl, min(x,y)=w360:dbl)
                n240 = property on="ROI" class="Bool (严格)"("Value"=FALSE ("ROI")) -> ()  [unwired: 2 in, 2 out]
                n241 = property on="X_start" class="DigNum (严格)"("Value"=w363) -> ()  [unwired: 2 in, 2 out]
                n242 = property on="Y_start" class="DigNum (严格)"("Value"=w360) -> ()  [unwired: 2 in, 2 out]
                n243 = property on="X_end" class="DigNum (严格)"("Value"=w362) -> ()  [unwired: 2 in, 2 out]
                n244 = property on="Y_end" class="DigNum (严格)"("Value"=w361) -> ()  [unwired: 2 in, 2 out]
              }
              frame False {
                w379 = 0.0 ("f")
                # "zoom view"
                n245 = Greater?(x=w371, y=w370) -> (0:w384:cluster{"X":bool, "Y":bool})
                n246 = Unbundle(w371) -> ("X"=w373:dbl, "Y"=w372:dbl)
                n247 = Unbundle(w370) -> ("X"=w375:dbl, "Y"=w374:dbl)
                n248 = Unbundle(w384) -> ("X"=w383:bool, "Y"=w382:bool)
                n249 = Select(t=1.0, s=w383, f=w379) -> (s? t:f=w378:dbl)
                n250 = Select(t=2.0, s=w382, f=w379) -> (s? t:f=w377:dbl)
                n251 = Add(x=w378, y=w377) -> (x+y=w376:dbl)
                n252 = case shown="0, 默认" w376 {
                  tunnel: w375 -> [_ _ _ w390]
                  tunnel: w374 -> [_ _ _ w389]
                  tunnel: w373 -> [_ _ _ w388]
                  tunnel: w372 -> [_ _ _ w387]
                  frame 0, Default {
                    w385 = u16 512 ("disp_xe")
                    w386 = u16 1 ("disp_xs")
                    n253 = local write "disp_xe"(w385) -> ()
                    n254 = local write "disp_xs"(w386) -> ()
                    n255 = local write "disp_ye"(w385) -> ()
                    n256 = local write "disp_ys"(w386) -> ()
                  }
                  frame 1 {
                  }
                  frame 2 {
                  }
                  frame 3 {
                    n257 = local write "disp_xs"(w390) -> ()
                    n258 = local write "disp_xe"(w388) -> ()
                    n259 = local write "disp_ys"(w389) -> ()
                    n260 = local write "disp_ye"(w387) -> ()
                  }
                }
              }
            }
          }
        }
      }
      event "MotorMgr": Value Change {
        n261 = event-data() -> ("NewVal"=w393:bool)  [unwired: 1 in, 4 out]
        n262 = vi-ref "ctrlMain.vi"() -> (w392:refnum<vi>)
        n263 = case shown="真" w393 {
          tunnel: w392 -> [w396 w403]
          tunnel: [w394 w397] -> w391
          frame False {
            n264 = invoke class="VI" method="Abort VI"(reference=w396) -> (reference out=w395:refnum<vi>)  [unwired: 2 in, 2 out]
            n265 = invoke class="VI" method="FP.Close"(reference=w395) -> (reference out=w394:refnum<vi>)  [unwired: 2 in, 2 out]
          }
          frame True {
            n266 = invoke class="VI" method="Run VI"(reference=w403, "Wait until done"=FALSE ("结束前等待"), "Auto Dispose Ref"=TRUE ("自动销毁引用")) -> (reference out=w400:refnum<vi>)  [unwired: 2 in, 4 out]
            n267 = invoke class="VI" method="FP.Open"(reference=w400, "Activate"=TRUE ("激活？"), "State"=T10."Standard" ("状态")) -> (reference out=w397:refnum<vi>)  [unwired: 2 in, 4 out]
          }
        }
        n268 = Close Reference(reference=w391) -> ()  [unwired: 1 in, 1 out]
      }
      event "Scan": Value Change {
        n269 = event-data() -> ("NewVal"=w406:bool)  [unwired: 1 in, 4 out]
        n270 = vi-ref "scanTest.vi"() -> (w405:refnum<vi>)
        n271 = case shown="真" w406 {
          tunnel: w405 -> [w409 w416]
          tunnel: [w407 w410] -> w404
          frame False {
            n272 = invoke class="VI" method="Abort VI"(reference=w409) -> (reference out=w408:refnum<vi>)  [unwired: 2 in, 2 out]
            n273 = invoke class="VI" method="FP.Close"(reference=w408) -> (reference out=w407:refnum<vi>)  [unwired: 2 in, 2 out]
          }
          frame True {
            n274 = invoke class="VI" method="FP.Open"(reference=w416, "Activate"=TRUE ("激活？"), "State"=T10."Standard" ("状态")) -> (reference out=w413:refnum<vi>)  [unwired: 2 in, 4 out]
            n275 = invoke class="VI" method="Run VI"(reference=w413, "Wait until done"=FALSE ("结束前等待"), "Auto Dispose Ref"=TRUE ("自动销毁引用")) -> (reference out=w410:refnum<vi>)  [unwired: 2 in, 4 out]
          }
        }
        n276 = Close Reference(reference=w404) -> ()  [unwired: 1 in, 1 out]
      }
      event "Analysis": Value Change {
        n277 = event-data() -> ("NewVal"=w419:bool)  [unwired: 1 in, 4 out]
        n278 = vi-ref "AnalysisPannel.vi"() -> (w418:refnum<vi>)
        n279 = case shown="真" w419 {
          tunnel: w418 -> [w422 w429]
          tunnel: [w420 w423] -> w417
          frame False {
            n280 = invoke class="VI" method="Abort VI"(reference=w422) -> (reference out=w421:refnum<vi>)  [unwired: 2 in, 2 out]
            n281 = invoke class="VI" method="FP.Close"(reference=w421) -> (reference out=w420:refnum<vi>)  [unwired: 2 in, 2 out]
          }
          frame True {
            n282 = invoke class="VI" method="FP.Open"(reference=w429, "Activate"=TRUE ("激活？"), "State"=T10."Standard" ("状态")) -> (reference out=w426:refnum<vi>)  [unwired: 2 in, 4 out]
            n283 = invoke class="VI" method="Run VI"(reference=w426, "Wait until done"=FALSE ("结束前等待"), "Auto Dispose Ref"=TRUE ("自动销毁引用")) -> (reference out=w423:refnum<vi>)  [unwired: 2 in, 4 out]
          }
        }
        n284 = Close Reference(reference=w417) -> ()  [unwired: 1 in, 1 out]
      }
    }
    n285 = local read "close"() -> (w334:bool)
  }
